vi "LS_372_read_PID_parameters.vi"(5 "VISA-Ressourcenname (in)":refnum<visa-resource-name>, 6 "Temperature":dbl, 7 "error in (no error)":errorcluster caption="Fehler (Eingang, kein Fehler)") -> (0 "Gain (P)":dbl, 1 "Reset (I)":dbl, 2 "Rate (D)":dbl, 3 "error out":errorcluster caption="Fehler (Ausgang)", 4 "VISA-Ressourcenname (out)":refnum<visa-resource-name>)   [LabVIEW 2018]
panel:
  out "upper temperature limit":dbl
  out "Heater Table parameter":string(combo)
  out "String":string
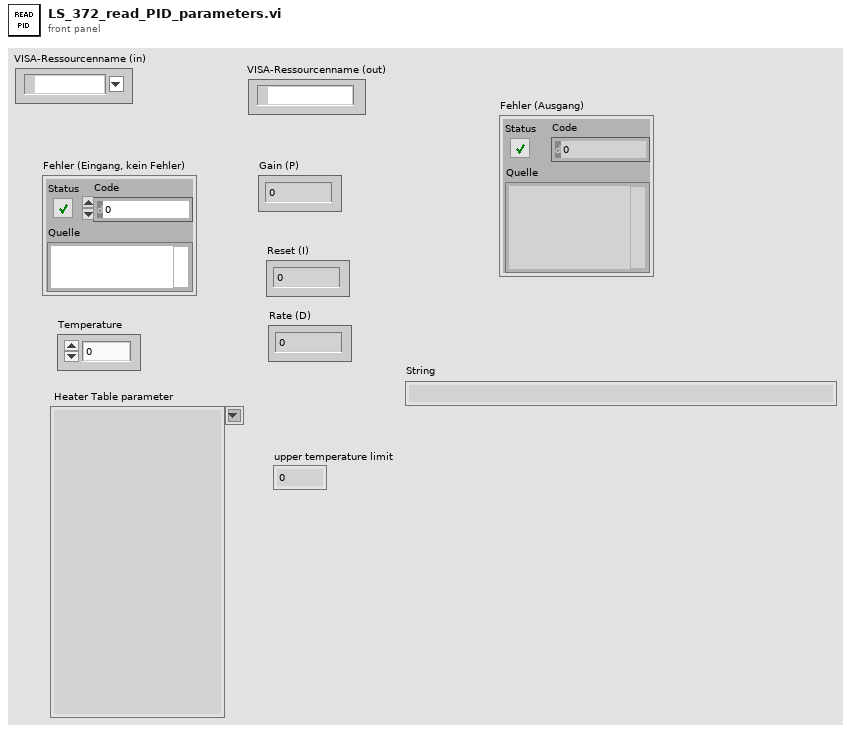
[diagram p1: front panel]
types:
  T1 = enum16{"open", "replace", "create", "open or create", "replace or create", "replace or create with confirmation"}
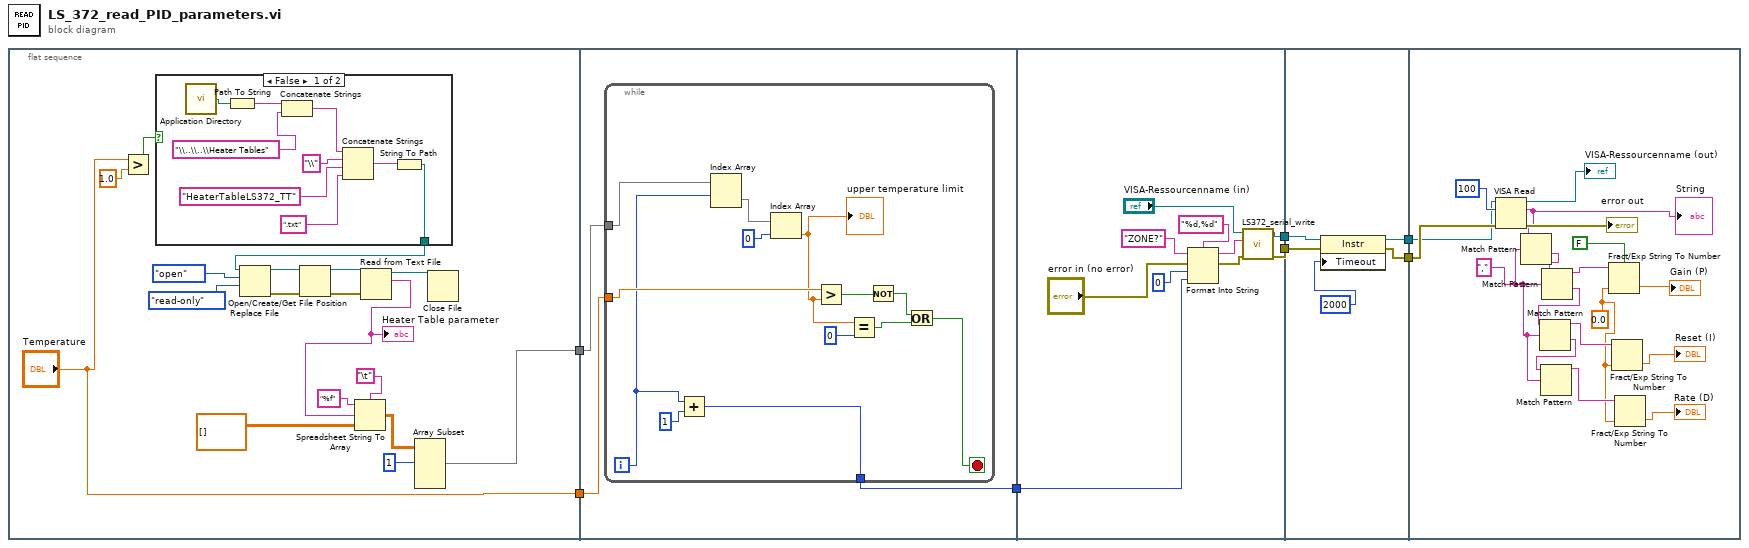
[diagram p0: block diagram]
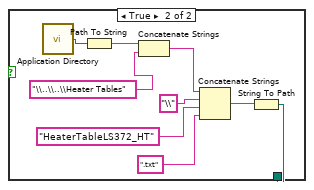
[diagram p2: hidden frame]
diagram:
  n1 = flat-sequence {
    tunnel: [w9] -> w3
    tunnel: ["Temperature"] -> w2
    tunnel: w3 -> [w46]
    tunnel: w2 -> [w45]
    tunnel: [w44] -> w1
    tunnel: [w68] -> w7
    tunnel: [w67] -> w6
    tunnel: w1 -> [w60]
    tunnel: w7 -> [w74]
    tunnel: w6 -> [w73]
    tunnel: [w71] -> w5
    tunnel: [w70] -> w4
    tunnel: w5 -> [w90]
    tunnel: w4 -> [w92]
    frame #0 {
      n2 = Greater?(x="Temperature", y=1.0) -> (0:w25:bool)
      n3 = case shown="False" w25 {
        tunnel: [w26 w35] -> w16
        frame False {
          n4 = call <vilib>:"Application Directory.vi"() -> ("Application Directory"=w34:path)
          n5 = Path To String(path=w34) -> (string=w33:string)
          n6 = Concatenate Strings(w33, "\\..\\..\\Heater Tables") -> (w31:string)
          n7 = Concatenate Strings(w31, "\\", "HeaterTableLS372_TT", ".txt") -> (w27:string)
          n8 = String To Path(string=w27) -> (path=w26:path)
        }
        frame True {
          n9 = call <vilib>:"Application Directory.vi"() -> ("Application Directory"=w43:path)
          n10 = Path To String(path=w43) -> (string=w42:string)
          n11 = Concatenate Strings(w42, "\\..\\..\\Heater Tables") -> (w40:string)
          n12 = Concatenate Strings(w40, "\\", "HeaterTableLS372_HT", ".txt") -> (w36:string)
          n13 = String To Path(string=w36) -> (path=w35:path)
        }
      }
      n14 = Open/Create/Replace File(file path (use dialog)=w16, operation (0:open)=T1."open", access (0:read/write)=enum16{"read/write", "read-only", "write-only"}."read-only") -> (refnum out=w21:refnum<file>, error out=w20:errorcluster)  [unwired: 3 in, 1 out]
      n15 = Get File Position(4:w20, 7:w21) -> (0:w18:errorcluster, 3:w19:refnum<file>)  [unwired: 1 out]
      n16 = Read from Text File(file (use dialog)=w19, error in=w18) -> (refnum out=w17:refnum<file>, text=w13:string)  [unwired: 2 in, 2 out]
      "Heater Table parameter" <- w13
      n17 = Spreadsheet String To Array(delimiter (Tab)="\t", format string="%f", spreadsheet string=w13, array type (2D Dbl)=dbl[][] []) -> (array=w11:dbl[][])
      n18 = Array Subset(array=w11, index (row)=1) -> (w9:dbl[][])  [unwired: 3 in]
      n19 = Close File(refnum=w17) -> ()  [unwired: 1 in, 2 out]
    }
    frame #1 {
      n20 = while {
        tunnel: w46 -> [w59]
        tunnel: w45 -> [w56]
        tunnel: [w47] -> w44
        i -> [w48]
        stop <- w51 stop-if-true
        n21 = Add(x=w48, y=1) -> (x+y=w47:i32)
        n22 = Index Array(array=w59, index (row)=w48) -> (element=w58:dbl[])  [unwired: 1 in]
        n23 = Index Array(array=w58, index=0) -> (element=w50:dbl)
        "upper temperature limit" <- w50
        n24 = Greater?(x=w56, y=w50) -> (0:w54:bool)
        n25 = Equal?(x=w50, y=0) -> (x = y?=w52:bool)
        n26 = Not(x=w54) -> (.not. x?=w53:bool)
        n27 = Or(x=w53, y=w52) -> (x .or. y?=w51:bool)
      }
    }
    frame #2 {
      n28 = Format Into String(format string="%d,%d", initial string="ZONE?", error in="error in (no error)", 0, w60) -> (resulting string=w63:string, error out=w61:errorcluster)
      n29 = call "LS372_serial_write.vi"("error in (no error)"=w61, "Write Buffer (\"\")"=w63, "VISA resource name"="VISA-Ressourcenname (in)") -> ("error out"=w67:errorcluster, "VISA resource name out"=w68:refnum<visa-resource-name>)  [unwired: 6 in, 1 out]
    }
    frame #3 {
      n30 = property class="Instr"(reference=w74, error in=w73, "Timeout"=2000) -> (reference out=w71:refnum<visa-resource-name>, error out=w70:errorcluster)
    }
    frame #4 {
      w81 = 0.0
      w77 = ","
      n31 = VISA Read(VISA resource name=w90, byte count=100, error in (no error)=w92) -> (VISA resource name out=→"VISA-Ressourcenname (out)":refnum<visa-resource-name>, read buffer=w75:string, error out=→"error out":errorcluster)  [unwired: 1 out]
      "String" <- w75
      n32 = Match Pattern(string=w75, regular expression=w77) -> (after substring=w76:string)  [unwired: 1 in, 3 out]
      n33 = Match Pattern(string=w76, regular expression=w77) -> (before substring=w78:string, after substring=w85:string)  [unwired: 1 in, 2 out]
      n34 = Match Pattern(string=w85, regular expression=w77) -> (before substring=w84:string, after substring=w83:string)  [unwired: 1 in, 2 out]
      n35 = Match Pattern(string=w83, regular expression=w77) -> (before substring=w82:string)  [unwired: 1 in, 3 out]
      n36 = Fract/Exp String To Number(use system decimal point (T)=FALSE, string=w78, default (0 dbl)=w81) -> (number=→"Gain (P)":dbl)  [unwired: 1 in, 1 out]
      n37 = Fract/Exp String To Number(string=w84, default (0 dbl)=w81) -> (number=→"Reset (I)":dbl)  [unwired: 2 in, 1 out]
      n38 = Fract/Exp String To Number(string=w82, default (0 dbl)=w81) -> (number=→"Rate (D)":dbl)  [unwired: 2 in, 1 out]
    }
  }
